vi "jt_analysis_from_master_log.vi"(9 "Experiment Indicator":string, 11 "Master log filepath":path) -> ()   [LabVIEW 2016]
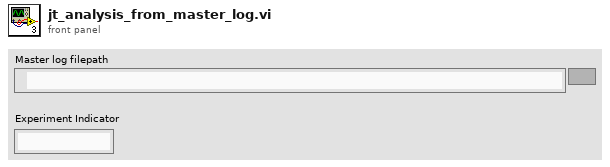
[diagram p1: front panel]
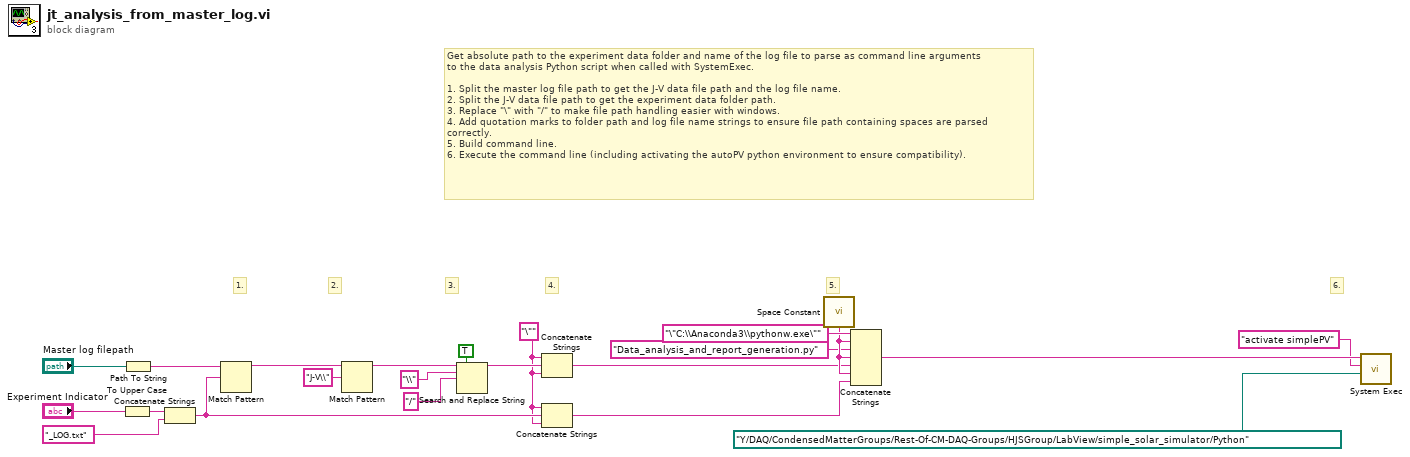
[diagram p0: block diagram]
diagram:
  w5 = "\"" ("string")
  # "6."
  # "5."
  # "4."
  # "3."
  # "2."
  # "1."
  # "Get absolute path to the experiment data folder and name of the log file to parse as command line arguments\nto the data analysis Python script when called with SystemExec.\n\n1. Split the master log file path to get the J-V data file path and the log file name.\n2. Split the J-V data file path to get the experiment data folder path.\n3. Replace \"\\\" with \"/\" to make file path handling easier with windows.\n4. Add quotation marks to folder path and log file name strings to ensure file path containing spaces are parsed\ncorrectly.\n5. Build command line.\n6. Execute the command line (including activating the autoPV python environment to ensure compatibility)."
  n1 = To Upper Case(1:"Experiment Indicator") -> (0:w20:string)
  n2 = Path To String(path="Master log filepath") -> (string=w15:string)
  n3 = Concatenate Strings(w20, "_LOG.txt") -> (w16:string)
  n4 = Match Pattern(string=w15, regular expression=w16) -> (before substring=w11:string)  [unwired: 1 in, 3 out]
  n5 = Match Pattern(string=w11, regular expression="J-V\\") -> (before substring=w10:string)  [unwired: 1 in, 3 out]
  n6 = Search and Replace String(replace all?=TRUE ("replace all? (F)"), input string=w10, search string="\\", replace string="/" ("search string")) -> (result string=w14:string)  [unwired: 4 in, 3 out]
  n7 = Concatenate Strings(w5, w14, w5) -> (w4:string)
  n8 = Concatenate Strings(w5, w16, w5) -> (w3:string)
  n9 = call <vilib>:"Space Constant.vi"() -> ("String"=w7:string)
  n10 = Concatenate Strings("\"C:\\Anaconda3\\pythonw.exe\"" ("string"), w7, "Data_analysis_and_report_generation.py" ("string"), w7, w4, w7, w3) -> (w2:string)
  n11 = call <vilib>:"System Exec.vi"("working directory"=path "Y:/DAQ/CondensedMatterGroups/Rest-Of-CM-DAQ-Groups/HJSGroup/LabView/simple_solar_simulator/Python", "standard input"="activate simplePV", "command line"=w2) -> ()  [unwired: 5 in, 4 out]
